vi "Verify Coast to 0 time.vi"(0 "GEA2 Reference In":refnum<k24>, 11 "Error In":errorcluster) -> (4 "GEA2 Reference Out":refnum<k24>, 6 "Coast Pass/Fail":bool, 8 "Report Text":string, 15 "Error Out":errorcluster)   [LabVIEW 2016, in "TL27.lvlib"]
doc: "This vi can be used to read ERD every 1 sec for user selected repeat counts."
uses:
  Projects/TL27.lvlib
  C:/Automation/DLLs/PC Dot Net/GeaCommunication.dll
  Common/LabVIEW GEA2 Toolkit/LabVIEW_GEA2_Toolkit.lvlibp/type defs/Source_Destination.ctl
  Common/LabVIEW GEA2 Toolkit/LabVIEW_GEA2_Toolkit.lvlibp/type defs/ERD Read Data In.ctl
  Common/LabVIEW GEA2 Toolkit/LabVIEW_GEA2_Toolkit.lvlibp/type defs/Data Type.ctl
  Common/LabVIEW GEA2 Toolkit/LabVIEW_GEA2_Toolkit.lvlibp
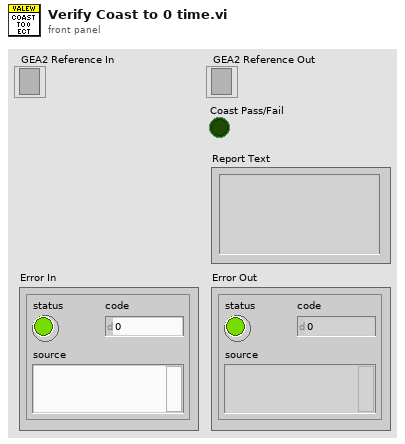
[diagram p1: front panel]
types:
  T1 = typedef "LabVIEW_GEA2_Toolkit.lvlibp/Source_Destination.ctl" = cluster{"Source":u8, "Destination":u8}
  T2 = typedef "LabVIEW_GEA2_Toolkit.lvlibp/ERD Read Data In.ctl" = cluster{"ERD Number":u16, "Data Type":T3}
  T3 = typedef "LabVIEW_GEA2_Toolkit.lvlibp/Data Type.ctl" = enum16{"string", "boolean", "uint8_t", "uint16_t", "uint32_t", "uint64_t", "int8_t", "int16_t", "int32_t", "int64_t"}
  T4 = enum16{"EQ (==)", "NE (!=)", "GT (>)", "LT (<)", "GE (>=)", "LE (<=)", "GTLT(> <)", "GELE (>= <=)", "GELT (>= <)", "GTLE (> <=)", "LTGT (< >)", "LEGE (<= >=)", "LEGT (<= >)", "LTGE (< >=)", "No Comparison"}
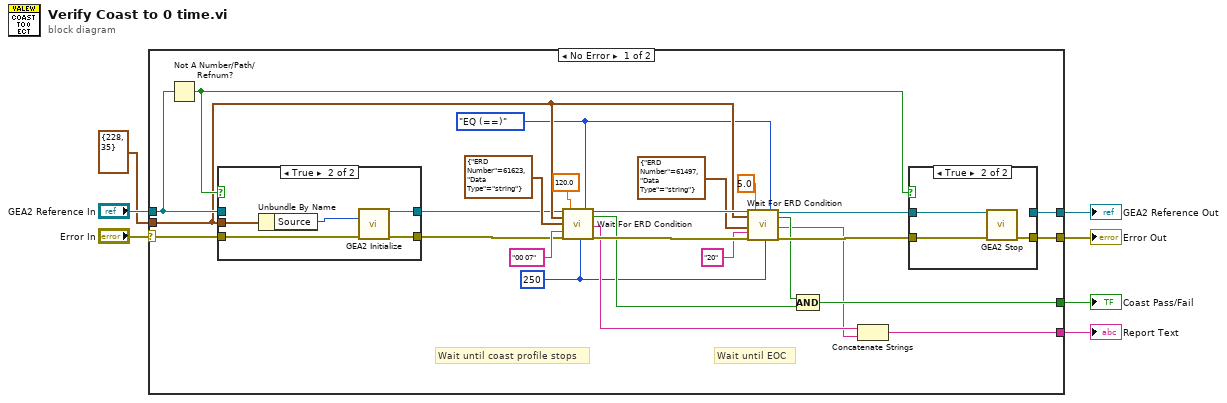
[diagram p0: block diagram]
diagram:
  n1 = case shown="No Error" "Error In" {
    selector: "Error In" -> [w32 w46]
    tunnel: T1 {"Source"=228, "Destination"=35} ("GEA Inputs") -> [w25 _]
    tunnel: "GEA2 Reference In" -> [w33 w47]
    tunnel: [w29 w47] -> w5
    tunnel: [w31 w46] -> w4
    tunnel: [w15 _] -> w2
    tunnel: [w12 _] -> w1
    frame No Error {
      w8 = u32 250 ("Loop Rate (ms)")
      w20 = T4."EQ (==)" ("Comparison")
      # "Wait until EOC"
      # "Wait until coast profile stops"
      n2 = Not A Number/Path/Refnum?(number/path/refnum=w33) -> (NaN/Path/Refnum?=w30:bool)
      n3 = case shown="True" w30 {
        tunnel: w32 -> [w40 w45]
        tunnel: [w40 w44] -> w9
        tunnel: [w39 w43] -> w10
        tunnel: w25 -> [_ w41]
        tunnel: w33 -> [w39 _]
        frame False {
        }
        frame True {
          n4 = Unbundle By Name(w41) -> ("Source"=w42:u8)
          n5 = call "GEA2 Initialize.vi"("Source Address"=w42, "error in"=w45) -> ("GEA2 Reference Out"=w43:refnum<k24>, "error out"=w44:errorcluster)  [unwired: 11 in, 1 out]
        }
      }
      n6 = call "Wait For ERD Condition.vi"("GEA2 Reference In"=w10, "GEA Inputs"=w25, "ERD Read Data"=T2 {"ERD Number"=61623, "Data Type"=enum."string"}, "Expected Low"="00 07" ("string"), "Error In"=w9, "Timeout (s)"=120.0, "Loop Rate (ms)"=w8, "Comparison"=w20) -> ("GEA2 Reference Out"=w26:refnum<k24>, "Pass/Fail?"=w16:bool, "Report Text"=w14:string, "Error Out"=w27:errorcluster)  [unwired: 7 in, 1 out]
      n7 = call "Wait For ERD Condition.vi"("GEA2 Reference In"=w26, "GEA Inputs"=w25, "ERD Read Data"=T2 {"ERD Number"=61497, "Data Type"=enum."string"}, "Expected Low"="20", "Error In"=w27, "Timeout (s)"=5.0, "Loop Rate (ms)"=w8, "Comparison"=w20) -> ("GEA2 Reference Out"=w19:refnum<k24>, "Pass/Fail?"=w17:bool, "Report Text"=w13:string, "Error Out"=w18:errorcluster)  [unwired: 7 in, 1 out]
      n8 = Compound Arithmetic op=AND(w17, w16) -> (w15:bool)
      n9 = Concatenate Strings(w14, w13) -> (w12:string)
      n10 = case shown="True" w30 {
        tunnel: [w34 w38] -> w31
        tunnel: w19 -> [w35 w37]
        tunnel: [w35 _] -> w29
        tunnel: w18 -> [w34 w36]
        frame False {
        }
        frame True {
          n11 = call "GEA2 Stop.vi"("GEA2 Reference In"=w37, "Error In"=w36) -> ("Error Out"=w38:errorcluster)  [unwired: 13 in]
        }
      }
    }
    frame Error {
    }
  }
  "GEA2 Reference Out" <- w5
  "Error Out" <- w4
  "Coast Pass/Fail" <- w2
  "Report Text" <- w1
